vi "ymode发送.vi"(2 "进度队列":refnum<queue>, 3 "硬件队列":refnum<queue>, 4 "硬件ID":refnum<k5>, 5 "文件（使用对话框）":path) -> ()   [LabVIEW 2015]
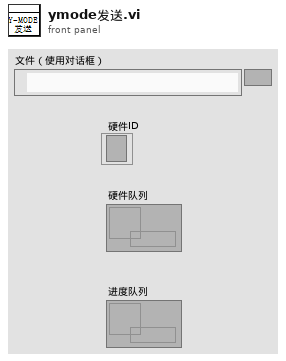
[diagram p1: front panel]
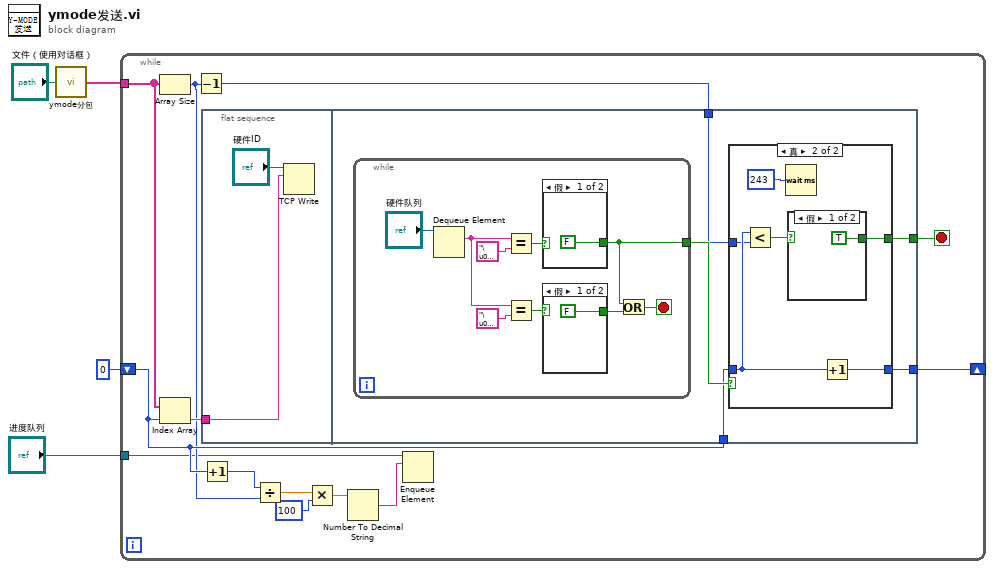
[diagram p0: block diagram]
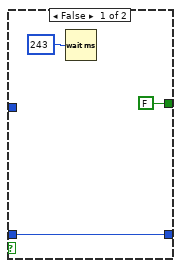
[diagram p2: hidden frame]
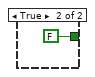
[diagram p3: hidden frame]
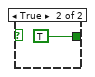
[diagram p4: hidden frame]
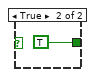
[diagram p5: hidden frame]
diagram:
  n1 = call "ymode分包.vi"("文件（使用对话框）"="文件（使用对话框）") -> ("分包数组"=w3:string[])
  n2 = while {
    tunnel: w3 -> [w15]
    shift-right: [w16] -> _
    shift-left: 0 -> [w12]
    tunnel: "进度队列" -> [w7]
    stop <- w14 stop-if-true
    n3 = Array Size(array=w15) -> (size(s)=w10:i32)
    n4 = Index Array(array=w15, index=w12) -> (element=w17:string)
    n5 = Decrement(x=w10) -> (x-1=w13:i32)
    n6 = flat-sequence {
      tunnel: w17 -> [w18]
      tunnel: w12 -> [w23]
      tunnel: [w22] -> w16
      tunnel: w13 -> [w21]
      tunnel: [w20] -> w14
      frame #0 {
        n7 = TCP Write(connection ID="硬件ID", data in=w18) -> ()  [unwired: 2 in, 3 out]
      }
      frame #1 {
        n8 = while {
          tunnel: [w36] -> w24
          stop <- w38 stop-if-true
          n9 = Dequeue Element(queue="硬件队列") -> (element=w40:string)  [unwired: 2 in, 3 out]
          n10 = Equal?(x=w40, y="\u0006") -> (x = y?=w42:bool)
          n11 = Equal?(x=w40, y="\u0015") -> (x = y?=w39:bool)
          n12 = case shown="假" w42 {
            tunnel: [FALSE TRUE] -> w36
            frame False {
            }
            frame True {
            }
          }
          n13 = case shown="假" w39 {
            tunnel: [FALSE TRUE] -> w37
            frame False {
            }
            frame True {
            }
          }
          n14 = Or(x=w36, y=w37) -> (x .or. y?=w38:bool)
        }
        n15 = case shown="真" w24 {
          tunnel: w23 -> [w27 w29]
          tunnel: [w27 w33] -> w22
          tunnel: w21 -> [_ w28]
          tunnel: [FALSE w30] -> w20
          frame False {
            n16 = Wait (ms)(milliseconds to wait=243) -> ()  [unwired: 1 out]
          }
          frame True {
            n17 = Less?(x=w29, y=w28) -> (x < y?=w31:bool)
            n18 = Wait (ms)(milliseconds to wait=243) -> ()  [unwired: 1 out]
            n19 = case shown="假" w31 {
              tunnel: [TRUE FALSE] -> w30
              frame False {
              }
              frame True {
              }
            }
            n20 = Increment(x=w29) -> (x+1=w33:i32)
          }
        }
      }
    }
    n21 = Increment(x=w12) -> (x+1=w11:i32)
    n22 = Divide(x=w11, y=w10) -> (x/y=w9:dbl)
    n23 = Multiply(x=w9, y=100) -> (x*y=w6:dbl)
    n24 = Number To Decimal String(number=w6) -> (decimal integer string=w5:string)  [unwired: 1 in]
    n25 = Enqueue Element(queue=w7, element=w5) -> ()  [unwired: 2 in, 3 out]
  }
